vi "FT_Set_Event_Notification.vi"(1 "EventHandle":i32, 2 "EventMask":u32(ring)=3 items=["FT_EVENT_RXCHAR"=1, "FT_EVENT_MODEM_STATUS"=2, "FT_EVENT_RXCHAR | FT_EVENT_MODEM_STATUS"=3], 3 "Handle":u32) -> (0 "FT_Status":u32(ring) items=["FT_OK", "FT_INVALID_HANDLE", "FT_DEVICE_NOT_FOUND", "FT_DEVICE_NOT_OPENED", "FT_IO_ERROR", "FT_INSUFFICIENT_RESOURCES", "FT_INVALID_PARAMETER", "FT_INVALID_BAUD_RATE", "FT_DEVICE_NOT_OPENED_FOR_ERASE", "FT_DEVICE_NOT_OPENED_FOR_WRITE", "FT_FAILED_TO_WRITE_DEVICE", "FT_EEPROM_READ_FAILED", "FT_EEPROM_WRITE_FAILED", "FT_EEPROM_ERASE_FAILED", "FT_EEPROM_NOT_PRESENT", "FT_EEPROM_NOT_PROGRAMMED", "FT_INVALID_ARGS", "FT_NOT_SUPPORTED", "FT_OTHER_ERROR"])   [LabVIEW 2019, in "D2XX.lvlib"]
uses:
  D2XX.lvlib
  FTD2XX.dll
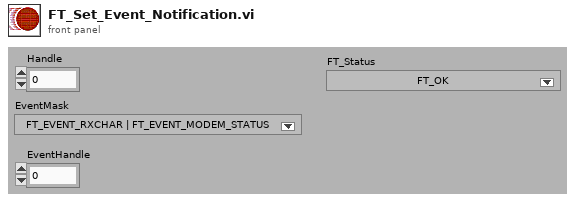
[diagram p1: front panel]
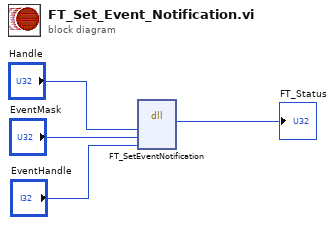
[diagram p0: block diagram]
diagram:
  n1 = dll-call lib="FTD2XX.dll" fn="FT_SetEventNotification"("Handle"="Handle", "EventMask"="EventMask", "pvArg"="EventHandle") -> ("FT_Status"=→"FT_Status":u32)  [unwired: 6 in, 2 out]
